vi "R-E Latch.vi"(1 "in":bool) -> (0 "out":bool)   [LabVIEW 2012]
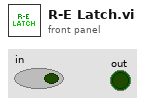
[diagram p1: front panel]
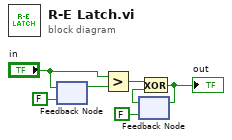
[diagram p0: block diagram]
diagram:
  n1 = feedback #1(FALSE) -> (w7:bool)
  n2 = feedback-in #1("in") -> ()
  n3 = Greater?(x="in", y=w7) -> (0:w5:bool)
  n4 = feedback #2(FALSE) -> (w4:bool)
  n5 = Exclusive Or(1:w4, 2:w5) -> (0:w2:bool)
  "out" <- w2
  n6 = feedback-in #2(w2) -> ()
